vi "sub_list cell color_rt.vi"(10 "millisecond timer":u32, 11 "sysTime":u32) -> (3 "cell color":u32(colorbox))   [LabVIEW 2011]
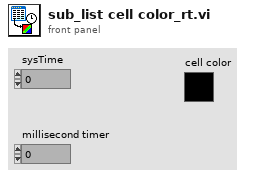
[diagram p1: front panel]
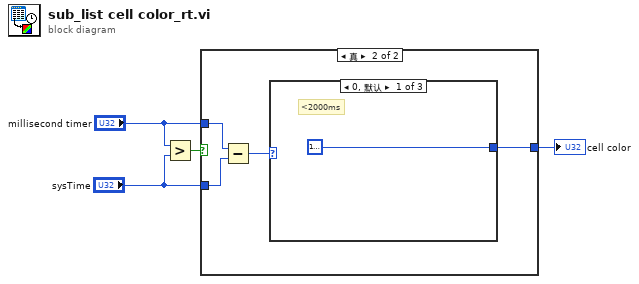
[diagram p0: block diagram]
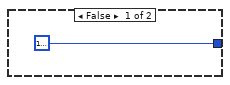
[diagram p2: hidden frame]
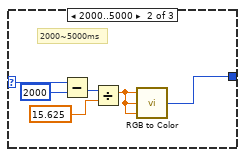
[diagram p3: hidden frame]
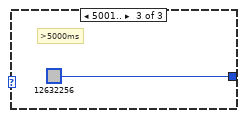
[diagram p4: hidden frame]
diagram:
  n1 = Greater?(x="millisecond timer", y="sysTime") -> (0:w4:bool)
  n2 = case shown="真" w4 {
    tunnel: "millisecond timer" -> [_ w9]
    tunnel: "sysTime" -> [_ w8]
    tunnel: [u32 16777222 w6] -> w1
    frame False {
    }
    frame True {
      n3 = Subtract(x=w9, y=w8) -> (x-y=w7:u32)
      n4 = case shown="0, 默认" w7 {
        selector: w7 -> [_ w16 _]
        tunnel: [u32 16777222 w11 u32 12632256] -> w6
        frame 0, Default {
          # "<2000ms"
        }
        frame 2000..5000 {
          # "2000~5000ms"
          n5 = Subtract(x=w16, y=u32 2000) -> (x-y=w14:u32)
          n6 = Divide(x=w14, y=15.625) -> (x/y=w12:dbl)
          n7 = call <vilib>:"RGB to Color.vi"("B"=w12, "G"=w12, "R"=w12) -> ("Color"=w11:u32)
        }
        frame 5001.. {
          # ">5000ms"
        }
      }
    }
  }
  "cell color" <- w1
